vi "iya.vi"() -> ()   [LabVIEW 2011]
panel:
  out "EX OR":bool
  in  "INPUT2 3":bool
  in  "INPUT1 3":bool
  out "NOR":bool
  in  "INPUT2 2":bool
  in  "INPUT1 2":bool
  out "NAND":bool
  in  "INPUT2":bool
  in  "INPUT1":bool
  out "NOT":bool
  in  "INPUT1":bool
  out "OR":bool
  in  "INPUT2":bool
  in  "INPUT1":bool
  out "AND":bool
  in  "INPUT 2":bool
  in  "INPUT1":bool
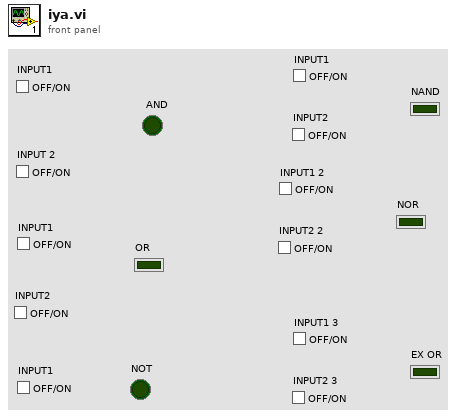
[diagram p1: front panel]
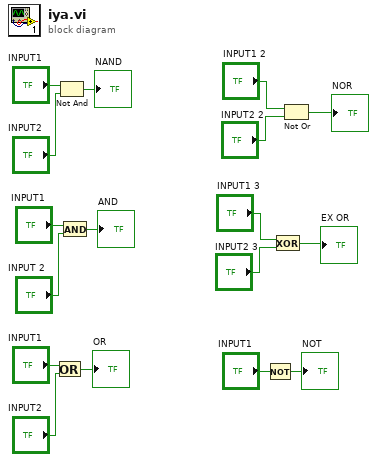
[diagram p0: block diagram]
diagram:
  n1 = Or(x="INPUT1", y="INPUT2") -> (x .or. y?=→"OR":bool)
  n2 = Not And(1:"INPUT2", 2:"INPUT1") -> (0:→"NAND":bool)
  n3 = And(x="INPUT1", y="INPUT 2") -> (x .and. y?=→"AND":bool)
  n4 = Not(x="INPUT1") -> (.not. x?=→"NOT":bool)
  n5 = Exclusive Or(1:"INPUT2 3", 2:"INPUT1 3") -> (0:→"EX OR":bool)
  n6 = Not Or(1:"INPUT2 2", 2:"INPUT1 2") -> (0:→"NOR":bool)
